vi "Receive and Prepare Messages.vi"(11 "Notifiers":T1) -> (0 "error out":errorcluster, 2 "params":variant, 3 "message":string)   [LabVIEW 2020]
uses:
  _Controls/Notifiers.ctl
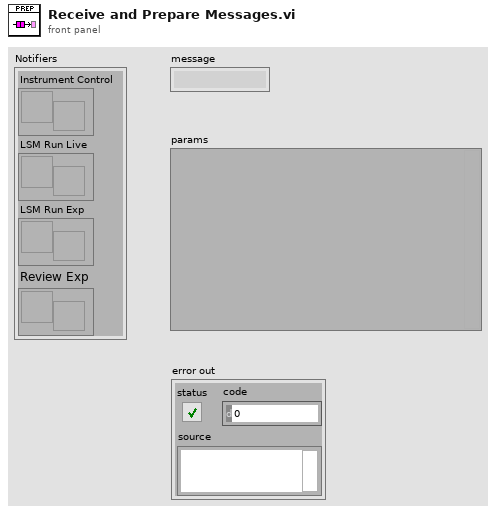
[diagram p1: front panel]
types:
  T1 = typedef "Notifiers.ctl" = cluster{"Instrument Control":refnum<notifier>, "LSM Run Live":refnum<notifier>, "LSM Run Exp":refnum<notifier>, "Review Exp":refnum<notifier>}
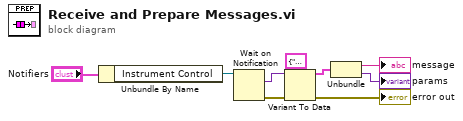
[diagram p0: block diagram]
diagram:
  n1 = Unbundle By Name("Notifiers") -> ("Instrument Control"=w2:refnum<notifier>)
  n2 = Wait on Notification(notifier=w2) -> (notification=w3:variant, error out=w5:errorcluster)  [unwired: 3 in, 2 out]
  n3 = Variant To Data(error in=w5, type=cluster{"message":string, "params":variant} {"message"="", "params"=variant} ("output cluster"), Variant=w3) -> (data=w4:cluster{"message":string, "params":variant}, error out=→"error out":errorcluster)
  n4 = Unbundle(w4) -> ("message"=→"message":string, "params"=→"params":variant)
